vi "Intake_execute.vi"   [LabVIEW 2020]
uses:
  <vilib>/Rock Robotics/WPI/Solenoid/WPI_SolenoidValue.ctl
  Globals/Intake_Globals.vi
types:
  T1 = typedef "WPI_SolenoidValue.ctl" = enum16{"Off", "On", "Forward", "Reverse"}
  T2 = typedef "Intake_cluster.ctl" = cluster{"control_states":T3, "%Vbus":dbl, "Trigger?":bool, "Manual_Extend?":bool, "Auto_Notifier":refnum<notifier>, "Step":dbl, "Parameter 1":dbl, "Parameter 2":dbl, "Parameter 3":dbl}
  T3 = typedef "Intake_control_states.ctl" = enum16{"No_Op", "Intake", "Manual", "Outtake", "Extend_No_Motor", "Retract_No_Motor"}
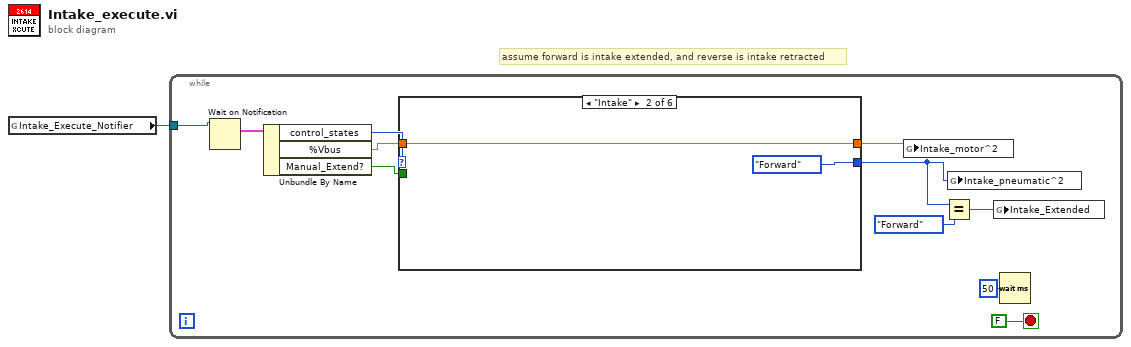
[diagram p0: block diagram]
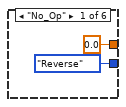
[diagram p2: hidden frame]
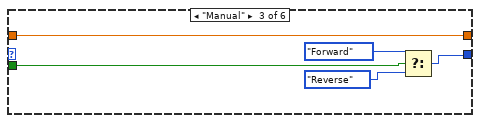
[diagram p3: hidden frame]
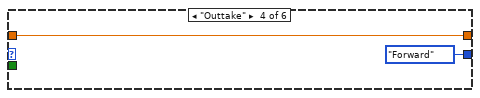
[diagram p4: hidden frame]
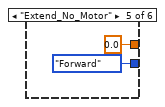
[diagram p5: hidden frame]
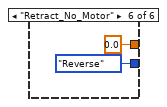
[diagram p6: hidden frame]
diagram:
  # "assume forward is intake extended, and reverse is intake retracted"
  n1 = global read "Intake_Globals.vi" "Intake_Execute_Notifier"() -> (w1:refnum<notifier>)
  n2 = while {
    tunnel: w1 -> [w12]
    stop <- FALSE stop-if-true
    n3 = Wait on Notification(notifier=w12) -> (notification=w9:T2)  [unwired: 3 in, 3 out]
    n4 = Unbundle By Name(w9) -> ("control_states"=w8:T3, "%Vbus"=w6:dbl, "Manual_Extend?"=w5:bool)
    n5 = case shown="\"Intake\"" w8 {
      tunnel: [0.0 ("Intake_motor^2") w15 w21 w22 0.0 ("%Vbus") 0.0 ("%Vbus")] -> w7
      tunnel: [WPI_SolenoidValue."Reverse" ("Value") WPI_SolenoidValue."Forward" ("Value") w17 WPI_SolenoidValue."Forward" ("Value") WPI_SolenoidValue."Forward" ("Value") WPI_SolenoidValue."Reverse" ("Value")] -> w4
      tunnel: w6 -> [_ w15 w21 w22 _ _]
      tunnel: w5 -> [_ _ w20 _ _ _]
      frame "No_Op" {
      }
      frame "Intake" {
      }
      frame "Manual" {
        n6 = Select(t=WPI_SolenoidValue."Forward" ("Value"), s=w20, f=WPI_SolenoidValue."Reverse" ("Value")) -> (s? t:f=w17:T1)
      }
      frame "Outtake" {
      }
      frame "Extend_No_Motor" {
      }
      frame "Retract_No_Motor" {
      }
    }
    n7 = global write "Intake_Globals.vi" "Intake_motor^2"(w7) -> ()
    n8 = Equal?(x=w4, y=WPI_SolenoidValue."Forward" ("Value")) -> (x = y?=w2:bool)
    n9 = global write "Intake_Globals.vi" "Intake_pneumatic^2"(w4) -> ()
    n10 = global write "Intake_Globals.vi" "Intake_Extended"(w2) -> ()
    n11 = Wait (ms)(milliseconds to wait=u32 50 ("millisecond timer value")) -> ()  [unwired: 1 out]
  }
